vi "Handle Mode.vi"(8 "error in (no error)":errorcluster, 11 "Stand in":refnum<class "Stand.lvclass">) -> (0 "error out":errorcluster, 3 "Stand out":refnum<class "Stand.lvclass">, 4 "dt ms handle mode":u32)   [LabVIEW 2019, in "Stand.lvclass"]
uses:
  Stand.lvclass
  D:/GIT H4000/H4000/src/Device_class/Device.lvclass
  Stand.lvclass/Stand.ctl
  TypeDef/Mode.ctl
  AI_class/AI.lvclass/AI.ctl
  AnalogComparator_class/AnalogComparator.lvclass/AnalogComparator.ctl
  Device_class/Device.lvclass/Device.ctl
  Valve_2DO_2DI_class/Valve_2DO_2DI.lvclass/Valve_2DO_2DI.ctl
  285b69a7-cd4c-45dd-8dd6-80699296fb4f.vi
  Nitro and Dut.vi
  Set Hi Press.vi
  AI_class/Get_Values.vi
  Invert Direction.vi
  Device_class/GetFPGA.vi
  Set Valve Mode.vi
  private/ExecuteStep.vi/d900ba76-673b-43eb-b747-4a40eb4a2de0.vi
  calc sp go up.vi/c91f4351-afbf-4a48-b204-0d489dec29b1.vi
  calc sp go up.vi/50fb84da-4633-4161-b856-f10d1b653a37.vi
  Valve_2DO_2DI_class/GetState.vi
  Valve_2DO_2DI_class/Open.vi
  Handle 44_1_2.vi/53daa488-cb92-467d-8939-09c81072894d.vi
  Handle 44_1_2.vi/27880750-5bda-4793-8800-8ef0418d5d30.vi
  Haskel Fast Forward.vi
  Set Hi Press.vi/29706e3b-acf2-4be0-8e3a-420f003c1de5.vi
  AnalogComparator_class/GetStatus.vi
  Valve State Mode.vi
  subvis/FastForward.vi
  Get U max Haskel.vi
  Get Accuracy.vi
  Valve State Mode.vi/810e184e-eeb6-4027-a8ae-1422f3ce3d45.vi
  Valve State Mode.vi/57bd4a65-f3dc-44f5-8d68-677c2a197570.vi
  Valve State Mode.vi/03b2f9e4-fceb-4725-9b90-3fd10082a088.vi
  Valve State Mode.vi/2785bab5-dd59-4d13-b638-b9157202fa4a.vi
  Valve State Mode.vi/50faa4b8-a9b4-4cc6-ab66-55c42b424fcd.vi
  Valve State Mode.vi/c882c3fe-b7a7-4419-8f9b-6788aa23338b.vi
  Valve State Mode.vi/3d0d09bd-48e8-482f-b1e2-a36b2bb65234.vi
  Valve State Mode.vi/33d3f26a-dc4a-4f56-bf0a-61d04c5d7434.vi
  Valve State Mode.vi/52af9d47-24d1-4057-80bf-8d93bfb3d17d.vi
  Valve State Mode.vi/bbc9916c-129f-4456-975e-9c3ae3d5db66.vi
  Valve State Mode.vi/a6106d78-2bf9-477e-b655-d47fad07ddfe.vi
  Valve State Mode.vi/e2916439-03c6-4471-bb40-42242a636e27.vi
  Valve State Mode.vi/094228cb-a119-423c-9af8-5a16f059a318.vi
  Valve State Mode.vi/bf5ad1e6-a0ae-4579-ad74-ca8f304cb7cf.vi
  Valve State Mode.vi/eb4d2b76-f0f0-4e1d-bda0-609c5f37b4e7.vi
  Valve_2DO_2DI_class/Valve_2DO_2DI.lvclass
  Global/Global Constant.vi
  private/Init Step.vi
  Set Backpressure.vi
  PreLoading.vi
  Const All Valve.vi
  <vilib>/addons/_JKI.lib/FPGA_Basic_Components/Counter JKI_FPGA.vi
  <vilib>/addons/_JKI.lib/FPGA_Basic_Components/Counter_32bit JKI_FPGA.vi
  NeedleValve_class/Do.vi
  private/Check Range Hi Press.vi
  Down Pressure.vi
  Set Ziro.vi
  Check Step is Done.vi
  PM_Group_class/All Stop.vi
  Valve_2DO_2DI_class/Close.vi
  FPGA_API_class/FPGA API.lvclass
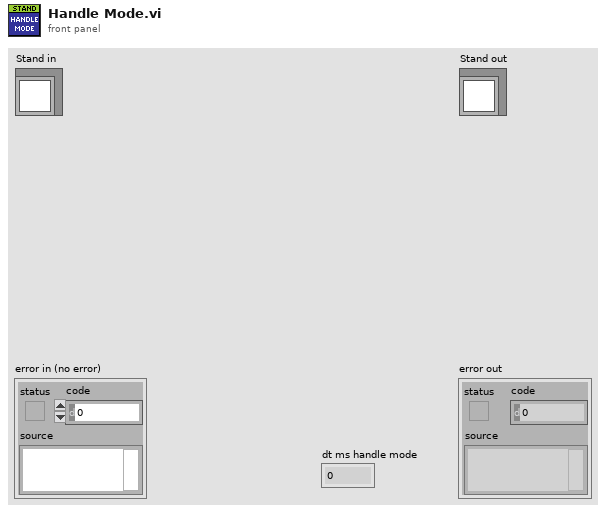
[diagram p1: front panel]
types:
  T1 = typedef "Mode.ctl" = enum16{"IDLE", "FILLING", "EXECUTE_SP", "DRAIN"}
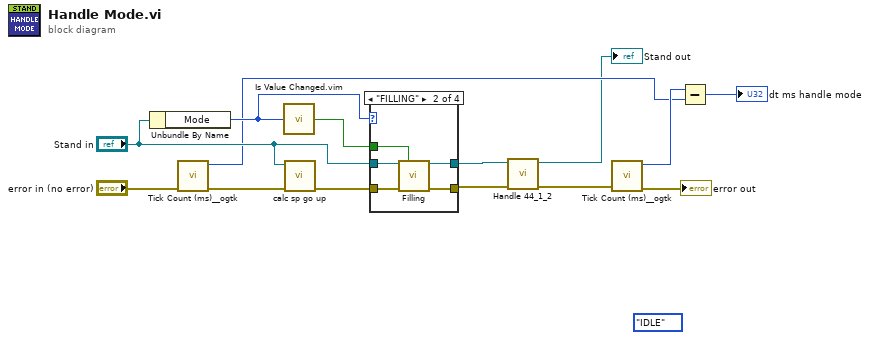
[diagram p0: block diagram]
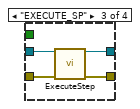
[diagram p3: hidden frame]
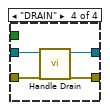
[diagram p4: hidden frame]
diagram:
  (unwired) Mode."IDLE" ("Data.Mode")
  n1 = Unbundle By Name("Stand in") -> ("Mode"=w14:T1)
  n2 = call <userlib>:"Tick Count (ms)__ogtk.vi"("error in (no error)"="error in (no error)") -> ("error out"=w9:errorcluster, "millisecond timer value"=w6:u32)  [unwired: 9 in]
  n3 = call "Is Value Changed.vim"("value"=w14) -> ("changed or first call?"=w13:bool)
  n4 = call "calc sp go up.vi"("error in (no error)"=w9, "Stand in"="Stand in") -> ("error out"=w11:errorcluster)  [unwired: 9 in]
  n5 = case shown="\"FILLING\"" w14 {
    tunnel: "Stand in" -> [w16 w21 w25 w29]
    tunnel: [w16 w18 w23 w26] -> w4
    tunnel: [w15 w19 w22 w27] -> w3
    tunnel: w11 -> [w15 w20 w24 w28]
    tunnel: w13 -> [_ w17 _ _]
    frame "IDLE" {
    }
    frame "FILLING" {
      n6 = call "Filling.vi"("reference in"=w21, "init"=w17, "error in (no error)"=w20) -> ("reference out"=w18:refnum<class "Stand.lvclass">, "error out"=w19:errorcluster)  [unwired: 11 in]
    }
    frame "EXECUTE_SP" {
      n7 = call "ExecuteStep.vi"("reference in"=w25, "error in (no error)"=w24) -> ("reference out"=w23:refnum<class "Stand.lvclass">, "error out"=w22:errorcluster)  [unwired: 12 in]
    }
    frame "DRAIN" {
      n8 = call "Handle Drain.vi"("error in (no error)"=w28, "Stand in"=w29) -> ("error out"=w27:errorcluster, "Stand out"=w26:refnum<class "Stand.lvclass">)  [unwired: 8 in]
    }
  }
  n9 = call "Handle 44_1_2.vi"("error in (no error)"=w3, "Stand in"=w4) -> ("error out"=w2:errorcluster, "Stand out"=→"Stand out":refnum<class "Stand.lvclass">)  [unwired: 8 in]
  n10 = call <userlib>:"Tick Count (ms)__ogtk.vi"("error in (no error)"=w2) -> ("error out"=→"error out":errorcluster, "millisecond timer value"=w7:u32)  [unwired: 9 in]
  n11 = Subtract(x=w7, y=w6) -> (x-y=→"dt ms handle mode":u32)
